vi "Write Experiment Parameters.vi"(8 "error in (no error)":errorcluster, 10 "Experiment Parameters":T1, 11 "SimpleExperimentService in":refnum<class "SimpleExperimentService.lvclass">) -> (0 "error out":errorcluster, 3 "SimpleExperimentService out":refnum<class "SimpleExperimentService.lvclass">)   [LabVIEW 2014]
uses:
  SimpleExperimentService.lvclass
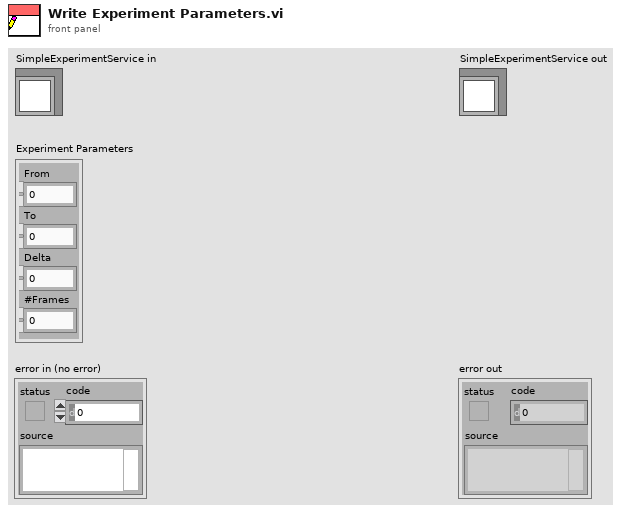
[diagram p1: front panel]
types:
  T1 = cluster{"From":dbl, "To":dbl, "Delta":dbl, "#Frames":u32}
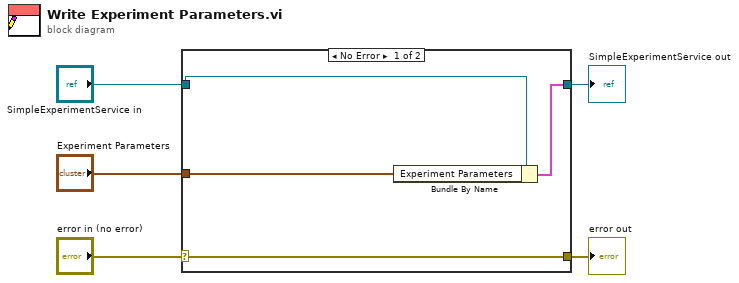
[diagram p0: block diagram]
diagram:
  n1 = case shown="No Error" "error in (no error)" {
    selector: "error in (no error)" -> [w9 w10]
    tunnel: [w9 w10] -> w4
    tunnel: [w7 w11] -> w2
    tunnel: "SimpleExperimentService in" -> [w8 w11]
    tunnel: "Experiment Parameters" -> [w6 _]
    frame No Error {
      n2 = Bundle By Name(cluster=w8, "Experiment Parameters"=w6) -> (w7:cluster{})
    }
    frame Error {
    }
  }
  "error out" <- w4
  "SimpleExperimentService out" <- w2
